vi "Config de Analogico.vi"(8 "error in":errorcluster, 10 "analogico":T1={"ANALOGICO CANALES"=[], "Numero de muestras"=1000, "Frecuencia de muestreo"=1000}) -> (0 "error out":errorcluster)   [LabVIEW 2020, in "Acquisition.lvlib"]
doc: "Manda la info que necesitamos para adquirir analogicamente \n_____\nCreated using Delacor QMH Event Scripter 6.0.0.121."
uses:
  Acquisition.lvlib
  cluster analogico.ctl
  Config de Analogico Argument--cluster.ctl
  CONTROLS.lvlib
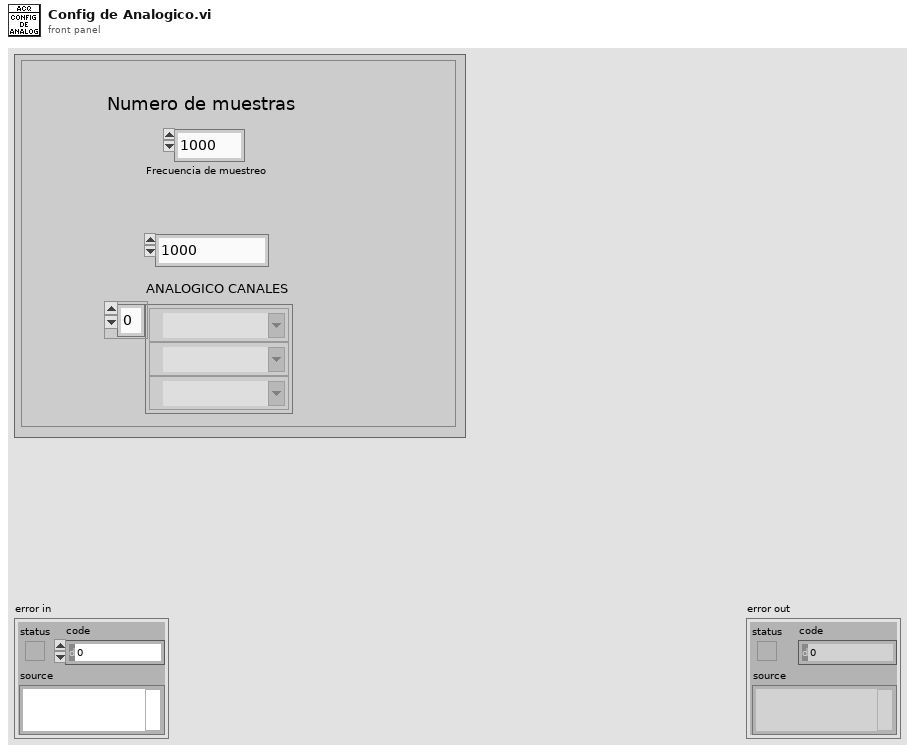
[diagram p1: front panel]
types:
  T1 = typedef "Acquisition.lvlib/CONTROLS.lvlib/cluster analogico.ctl" = cluster{"ANALOGICO CANALES":tag[], "Numero de muestras":u32, "Frecuencia de muestreo":u32}
  T2 = typedef "Acquisition.lvlib/Config de Analogico Argument--cluster.ctl" = cluster{"analogico":T1}
  T3 = typedef "Acquisition.lvlib/Request Events--cluster.ctl" = cluster{"Stop Module":refnum<user-event>, "Show Panel":refnum<user-event>, "Hide Panel":refnum<user-event>, "Get Module Execution Status":refnum<user-event>, "Show Diagram":refnum<user-event>, "Config de Analogico":refnum<user-event>, "Digital Parametros":refnum<user-event>}
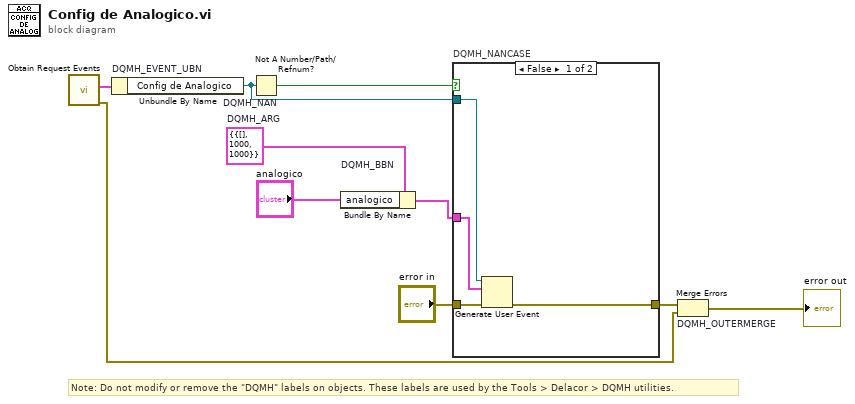
[diagram p0: block diagram]
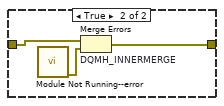
[diagram p2: hidden frame]
diagram:
  w4 = T2 {"analogico"={"ANALOGICO CANALES"=[], "Numero de muestras"=1000, "Frecuencia de muestreo"=1000}}  # DQMH_ARG
  # "Note: Do not modify or remove the \"DQMH\" labels on objects. These labels are used by the Tools > Delacor > DQMH utilities."
  n1 = call "Obtain Request Events.vi"() -> ("error out"=w2:errorcluster, "Acquisition Request Events"=w1:T3)  [unwired: 10 in]
  n2 = Unbundle By Name "DQMH_EVENT_UBN"(w1) -> ("Config de Analogico"=w6:refnum<user-event>)
  n3 = Not A Number/Path/Refnum? "DQMH_NAN"(number/path/refnum=w6) -> (NaN/Path/Refnum?=w7:bool)
  n4 = Bundle By Name "DQMH_BBN"(cluster=w4, "analogico"="analogico") -> (w8:T2)
  n5 = case "DQMH_NANCASE" shown="False" w7 {
    tunnel: "error in" -> [w14 w17]
    tunnel: [w13 w16] -> w5
    tunnel: w6 -> [w12 _]
    tunnel: w8 -> [w11 _]
    frame False {
      n6 = Generate User Event(user event=w12, event data cluster=w11, error in=w14) -> (error out=w13:errorcluster)  [unwired: 1 in, 1 out]
    }
    frame True {
      n7 = call "Module Not Running--error.vi"() -> ("error out"=w15:errorcluster)  [unwired: 11 in]
      n8 = Merge Errors "DQMH_INNERMERGE"(w17, w15) -> (w16:errorcluster)
    }
  }
  n9 = Merge Errors "DQMH_OUTERMERGE"(w5, w2) -> (→"error out":errorcluster)
